vi "Enable Disable Enum to Disabled.vi"(1 "Disabled":T1(ring)) -> (0 "Disabled":bool)   [LabVIEW 2018]
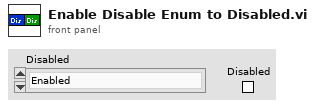
[diagram p1: front panel]
types:
  T1 = enum8{"Enabled", "Disabled", "Disabled and Grayed Out"}
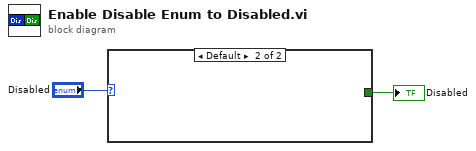
[diagram p0: block diagram]
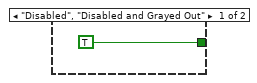
[diagram p2: hidden frame]
diagram:
  n1 = case shown="Default" "Disabled" {
    tunnel: [TRUE _] -> w1
    frame "Disabled", "Disabled and Grayed Out" {
    }
    frame Default {
    }
  }
  "Disabled" <- w1
